vi "Write limit_alarm_min.vi"(8 "error in (no error)":errorcluster caption="entrée d'erreur (pas d'erreur)", 10 "limit_alarm_min":dbl, 11 "DAQmxTaskAICurrent en entrée":refnum<class "DAQmxTaskAICurrent.lvclass">) -> (0 "error out":errorcluster caption="sortie d'erreur", 3 "DAQmxTaskAICurrent en sortie":refnum<class "DAQmxTaskAICurrent.lvclass">)   [LabVIEW 2015, in "DAQmxTaskAICurrent.lvclass"]
uses:
  DAQmxTaskAICurrent.lvclass
  DAQmxTaskAICurrent.lvclass/DAQmxTaskAICurrent.ctl
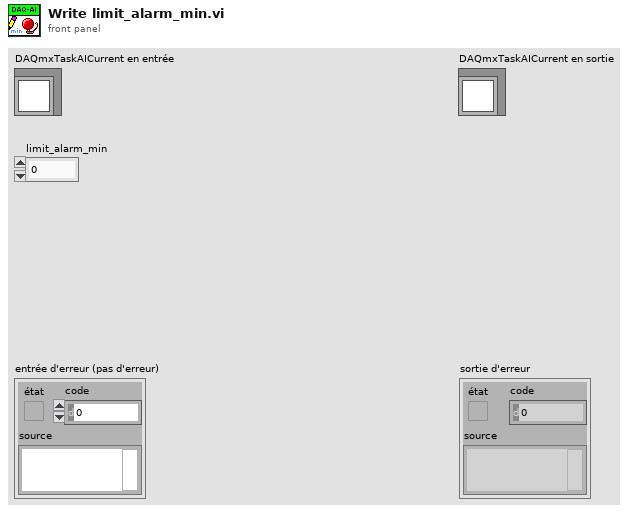
[diagram p1: front panel]
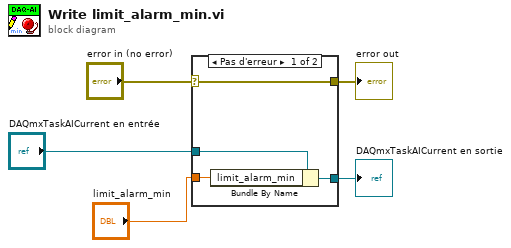
[diagram p0: block diagram]
diagram:
  n1 = case shown="Pas d'erreur" "error in (no error)" {
    selector: "error in (no error)" -> [w9 w10]
    tunnel: [w9 w10] -> w4
    tunnel: [w7 w11] -> w2
    tunnel: "DAQmxTaskAICurrent en entrée" -> [w8 w11]
    tunnel: "limit_alarm_min" -> [w6 _]
    frame No Error {
      n2 = Bundle By Name(cluster=w8, "limit_alarm_min"=w6) -> (w7:refnum<class "DAQmxTaskAICurrent.lvclass">)
    }
    frame Error {
    }
  }
  "error out" <- w4
  "DAQmxTaskAICurrent en sortie" <- w2
